vi "ControlsToCommands.vi"(11 "input cluster":T1) -> (3 "output cluster":T2)   [LabVIEW 2015]
uses:
  ControlsToCommands.ctl
  Controls.ctl
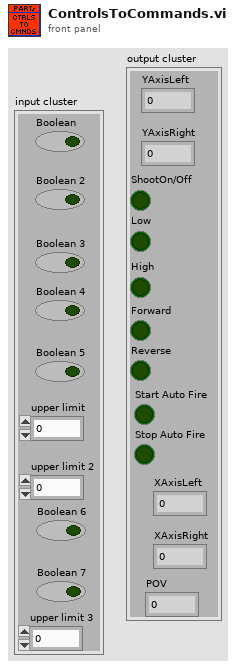
[diagram p1: front panel]
types:
  T1 = typedef "Controls.ctl" = cluster{"Boolean":bool, "Boolean 2":bool, "Boolean 3":bool, "Boolean 4":bool, "Boolean 5":bool, "upper limit":dbl, "upper limit 2":dbl, "Boolean 6":bool, "Boolean 7":bool, "upper limit 3":dbl}
  T2 = typedef "ControlsToCommands.ctl" = cluster{"YAxisLeft":dbl, "YAxisRight":dbl, "ShootOn/Off":bool, "Low":bool, "High":bool, "Forward":bool, "Reverse":bool, "Start Auto Fire":bool, "Stop Auto Fire":bool, "XAxisLeft":dbl, "XAxisRight":dbl, "POV":dbl}
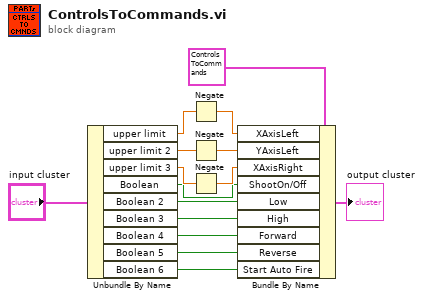
[diagram p0: block diagram]
diagram:
  n1 = Unbundle By Name("input cluster") -> ("upper limit"=w10:dbl, "upper limit 2"=w9:dbl, "upper limit 3"=w8:dbl, "Boolean"=w7:bool, "Boolean 2"=w6:bool, "Boolean 3"=w4:bool, "Boolean 4"=w5:bool, "Boolean 5"=w3:bool, "Boolean 6"=w2:bool)
  n2 = Negate(x=w10) -> (-x=w13:dbl)
  n3 = Negate(x=w9) -> (-x=w12:dbl)
  n4 = Negate(x=w8) -> (-x=w11:dbl)
  n5 = Bundle By Name(cluster=T2 {"YAxisLeft"=0.0, "YAxisRight"=0.0, "ShootOn/Off"=FALSE, "Low"=FALSE, "High"=FALSE, "Forward"=FALSE, "Reverse"=FALSE, "Start Auto Fire"=FALSE, "Stop Auto Fire"=FALSE, "XAxisLeft"=0.0, "XAxisRight"=0.0, "POV"=0.0} ("input cluster"), "XAxisLeft"=w13, "YAxisLeft"=w12, "XAxisRight"=w11, "ShootOn/Off"=w7, "Low"=w6, "High"=w4, "Forward"=w5, "Reverse"=w3, "Start Auto Fire"=w2) -> (→"output cluster":T2)
